vi "ex_Convert Array of Wfrms.vi"(1 "Array of Waveforms":waveform(dbl)[](array[waveform])) -> (0 "Last Element":dbl format="%0.2f")   [LabVIEW 2020]
doc: "Takes an array of waveforms as an input and returns the last element of the first waveform."
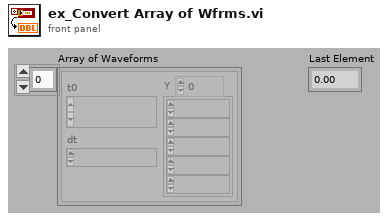
[diagram p1: front panel]
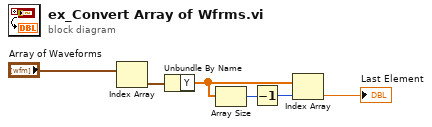
[diagram p0: block diagram]
diagram:
  n1 = Index Array(array="Array of Waveforms") -> (element=w5:waveform(dbl))  [unwired: 1 in]
  n2 = Unbundle By Name(w5) -> ("Y"=w4:dbl[])
  n3 = Array Size(array=w4) -> (size(s)=w3:i32)
  n4 = Decrement(x=w3) -> (x-1=w2:i32)
  n5 = Index Array(array=w4, index=w2) -> (element=→"Last Element":dbl)
